vi "SaveRoutine.vi"(0 "Path":path, 1 "No. of Assem":dbl, 2 "No. Pegs Rej":dbl, 3 "No. Rings Rej":dbl, 5 "No. Pegs":dbl, 7 "No. of Rings":dbl, 9 "No. RingQ":dbl, 12 "Total Rej":dbl, 13 "Rings Left":dbl, 14 "Pegs Left":dbl) -> ()   [LabVIEW 2016]
doc: "Saves an array of values to a file which was passed to it"
panel:
  in  "Time Target (s)":dbl=5.0
  out "Elapsed Time (s)":dbl
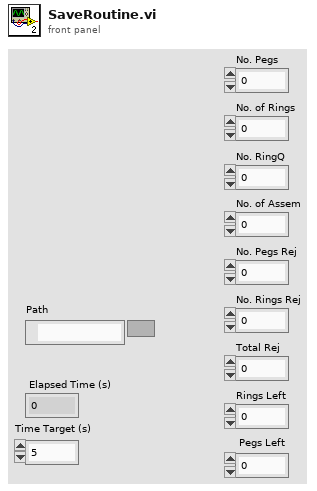
[diagram p1: front panel]
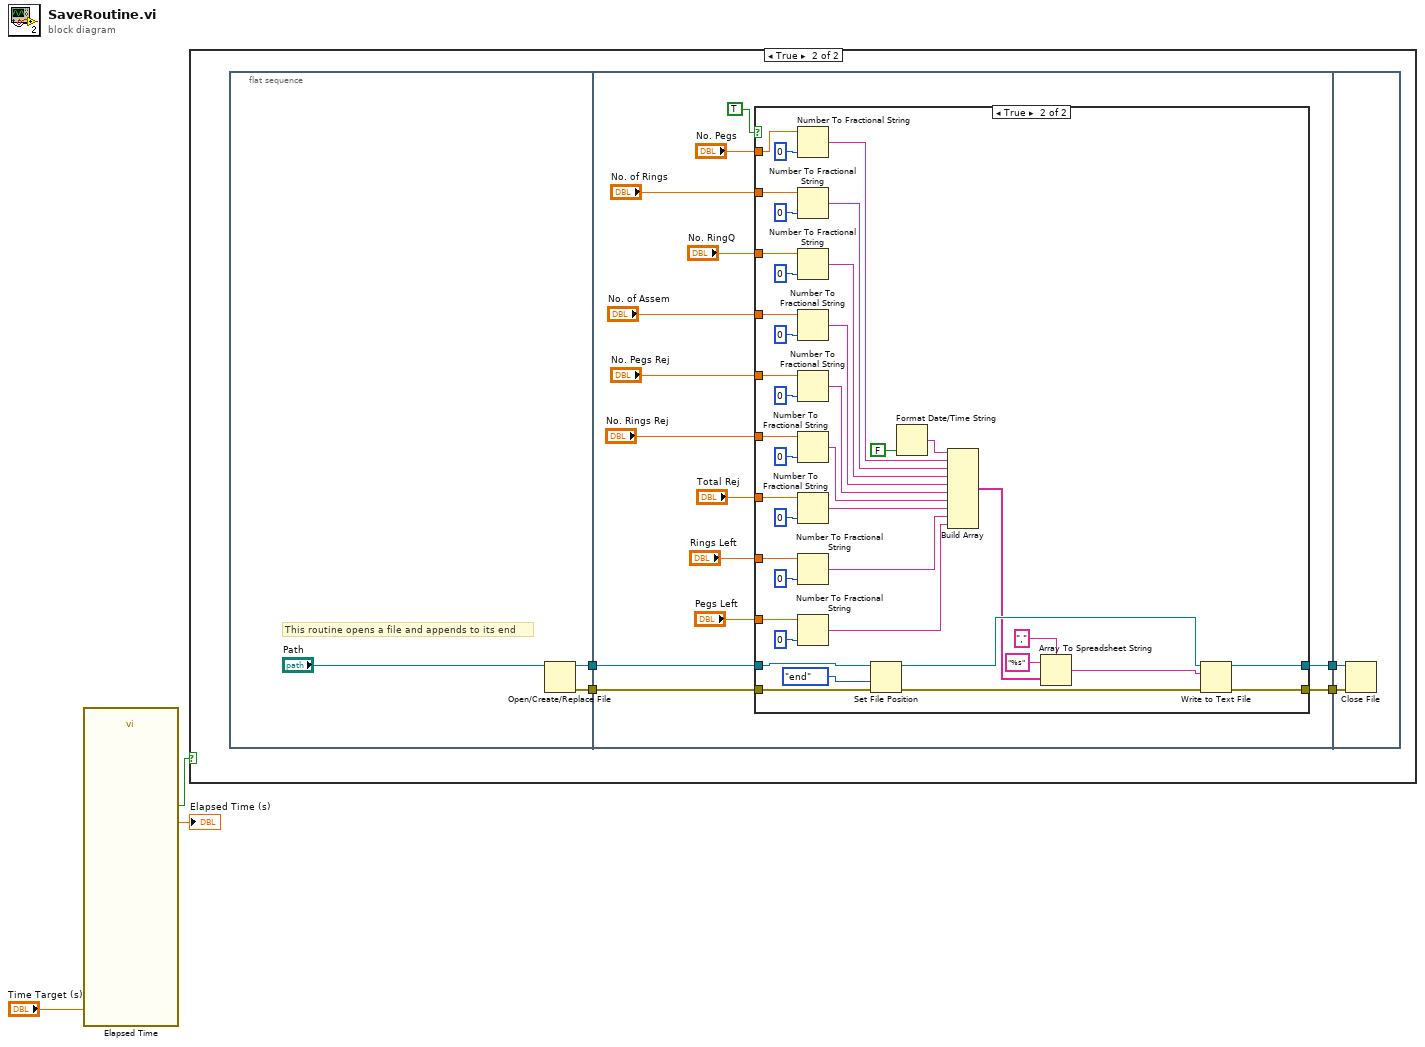
[diagram p0: block diagram]
diagram:
  n1 = call "Elapsed Time"("Time Target (s)"="Time Target (s)") -> ("Elapsed Time (s)"=→"Elapsed Time (s)":dbl, "Time has Elapsed"=w3:bool)  [unwired: 11 in, 6 out]
  n2 = case shown="True" w3 {
    frame False {
    }
    frame True {
      n3 = flat-sequence {
        tunnel: [w10] -> w7
        tunnel: [w9] -> w6
        tunnel: w7 -> [w15]
        tunnel: w6 -> [w14]
        tunnel: [w13] -> w5
        tunnel: [w12] -> w4
        tunnel: w5 -> [w68]
        tunnel: w4 -> [w67]
        frame #0 {
          # "This routine opens a file and appends to its end"
          n4 = Open/Create/Replace File(file path (use dialog)="Path") -> (refnum out=w10:refnum<file>, error out=w9:errorcluster)  [unwired: 5 in, 1 out]
        }
        frame #1 {
          n5 = case shown="True" TRUE {
            tunnel: [w26 w60] -> w13
            tunnel: "No. Pegs" -> [_ w42]
            tunnel: "Total Rej" -> [_ w41]
            tunnel: "No. Rings Rej" -> [_ w40]
            tunnel: "No. of Assem" -> [_ w39]
            tunnel: "No. RingQ" -> [_ w38]
            tunnel: "No. of Rings" -> [_ w37]
            tunnel: "Rings Left" -> [_ w36]
            tunnel: "Pegs Left" -> [_ w35]
            tunnel: "No. Pegs Rej" -> [_ w30]
            tunnel: [w25 w29] -> w12
            tunnel: w15 -> [w26 w28]
            tunnel: w14 -> [w25 w27]
            frame False {
            }
            frame True {
              n6 = Number To Fractional String(number=w42, precision (6)=i16 0) -> (F-format string=w45:string)  [unwired: 2 in]
              n7 = Number To Fractional String(number=w37, precision (6)=i16 0) -> (F-format string=w53:string)  [unwired: 2 in]
              n8 = Number To Fractional String(number=w38, precision (6)=i16 0) -> (F-format string=w54:string)  [unwired: 2 in]
              n9 = Number To Fractional String(number=w39, precision (6)=i16 0) -> (F-format string=w55:string)  [unwired: 2 in]
              n10 = Number To Fractional String(number=w30, precision (6)=i16 0) -> (F-format string=w56:string)  [unwired: 2 in]
              n11 = Number To Fractional String(number=w40, precision (6)=i16 0) -> (F-format string=w57:string)  [unwired: 2 in]
              n12 = Number To Fractional String(number=w41, precision (6)=i16 0) -> (F-format string=w58:string)  [unwired: 2 in]
              n13 = Number To Fractional String(number=w36, precision (6)=i16 0) -> (F-format string=w32:string)  [unwired: 2 in]
              n14 = Number To Fractional String(number=w35, precision (6)=i16 0) -> (F-format string=w31:string)  [unwired: 2 in]
              n15 = Set File Position(refnum=w28, from (0:start)=enum16{"start", "end", "current"}."end", error in=w27) -> (refnum out=w65:refnum<file>, error out=w64:errorcluster)  [unwired: 1 in]
              n16 = Format Date/Time String(UTC format=FALSE) -> (date/time string=w52:string)  [unwired: 2 in]
              n17 = Build Array(w52, w45, w53, w54, w55, w56, w57, w58, w32, w31) -> (w43:string[])
              n18 = Array To Spreadsheet String(delimiter (Tab)=",", array=w43, 3:"%s" ("format string")) -> (spreadsheet string=w63:string)
              n19 = Write to Text File(file (use dialog)=w65, text=w63, error in=w64) -> (refnum out=w60:refnum<file>, error out=w29:errorcluster)  [unwired: 1 in, 1 out]
            }
          }
        }
        frame #2 {
          n20 = Close File(refnum=w68, error in=w67) -> ()  [unwired: 2 out]
        }
      }
    }
  }
